vi "Create.vi"(8 "error in (no error)":errorcluster, 10 "JSON Builder (native)":refnum<class "JSON Builder.lvclass">, 11 "Configuration in":refnum<class "Configuration.lvclass">) -> (0 "error out":errorcluster, 3 "Configuration out":refnum<class "Configuration.lvclass">)   [LabVIEW 2017, in "DSF Core.lvlib" / "Configuration.lvclass"]
uses:
  Configuration.lvclass
  JSON Builder/JSON Builder.lvclass
  Configuration.lvclass/Configuration.ctl
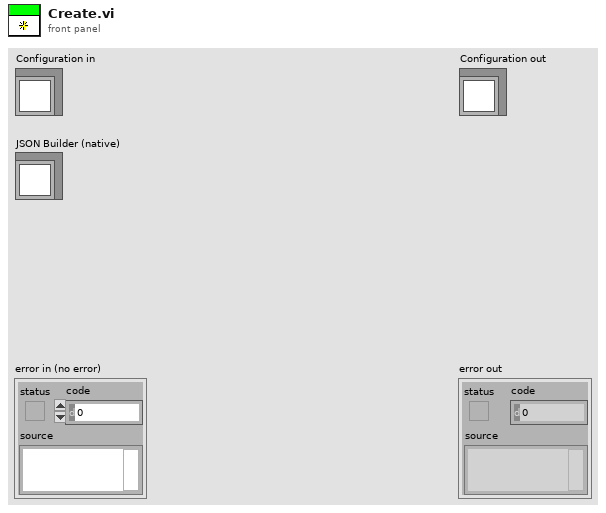
[diagram p1: front panel]
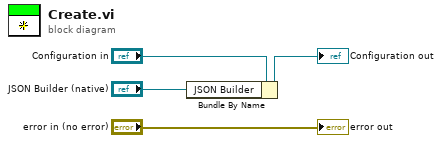
[diagram p0: block diagram]
diagram:
  n1 = Bundle By Name(cluster="Configuration in", "JSON Builder"="JSON Builder (native)") -> (→"Configuration out":refnum<class "Configuration.lvclass">)
  "error out" <- "error in (no error)"
